vi "Lab Panel V5.10.vi"() -> ()   [LabVIEW 2013] (continued)
                                n574 = TDMS Open(6:FALSE, 10:T20."create or replace" ("operation (0:open)"), 11:w887) -> (0:w886:errorcluster, 3:→"TDMS LAB01-2":refnum<k34>)  [unwired: 4 in]
                              }
                              frame #2 {
                                n575 = local read "SET LAB01-2"() -> (w897:T5)
                                n576 = local read "TDMS LAB01-2"() -> (w908:refnum<k34>)
                                n577 = Build Array("Testers Name", "Description", "Set Test Cycles", "T-Rise minutes", "T-Rise Deg C") -> (w898:string[])
                                n578 = Unbundle(w897) -> ("NAME"=w896:string, "DESCRIPTION"=w895:string, "CYCLES"=w894:dbl, "T-RISE mins"=w893:dbl, "T-RISE deg C"=w892:dbl)
                                n579 = Number To Decimal String(number=w894) -> (decimal integer string=w907:string)  [unwired: 1 in]
                                n580 = Number To Decimal String(number=w893) -> (decimal integer string=w906:string)  [unwired: 1 in]
                                n581 = Number To Decimal String(number=w892) -> (decimal integer string=w905:string)  [unwired: 1 in]
                                n582 = Build Array(w896, w895, w907, w906, w905) -> (w904:string[])
                                n583 = TDMS Set Properties(5:w904, 7:w898, 11:w908) -> ()  [unwired: 3 in, 4 out]
                              }
                              frame #3 {
                                n584 = local read "DISP LAB01-2"() -> (w910:T4)
                                n585 = Concatenate Strings("LAB01-2  ", w913) -> (w914:string)
                                n586 = Two Button Dialog(message=w914, 1:w911, 2:w912) -> (T button?=w916:bool)
                                n587 = case shown="True" w916 {
                                tunnel: w910 -> [w923 w924]
                                tunnel: [w923 w924] -> w920
                                tunnel: [w922 w925] -> w919
                                tunnel: [w921 w925] -> w918
                                frame False {
                                n588 = Unbundle(w923) -> ("CYCLE"=w922:dbl, "MINS"=w921:dbl)  [unwired: 1 out]
                                }
                                frame True {
                                w925 = 0.0
                                }
                                }
                                n589 = Bundle(cluster=w920, "CYCLE"=w919, "MINS"=w918, "STATUS"="RUN") -> (w909:T4)
                                n590 = local write "DISP LAB01-2"(w909) -> ()
                              }
                              frame #4 {
                                n591 = local read "TEMP START LAB01-2"() -> (w928:cluster{"TL":dbl, "TN":dbl})
                                n592 = Bundle(cluster=w928, "TL"=w926, "TN"=w926) -> (w927:cluster{"TL":dbl, "TN":dbl})
                                n593 = local write "TEMP START LAB01-2"(w927) -> ()
                              }
                            }
                          }
                        }
                      }
                    }
                  }
                }
              }
              event "RUN LAB02-1": Value Change {
                n594 = event-data() -> ("NewVal"=w934:bool)  [unwired: 1 in, 5 out]
                n595 = local read "SIG LAB02-1"() -> (w930:T2)
                n596 = case shown="True" w934 {
                  tunnel: w940 -> [_ w978]
                  tunnel: w939 -> [_ w977]
                  tunnel: w937 -> [w942 w976]
                  tunnel: w938 -> [_ w975]
                  tunnel: w936 -> [_ w974]
                  tunnel: [w941 w973] -> w935
                  tunnel: w933 -> [_ w972]
                  tunnel: w932 -> [_ w971]
                  tunnel: w931 -> [_ w970]
                  tunnel: w930 -> [_ w969]
                  tunnel: w929 -> [_ w968]
                  frame False {
                    # "stop test"
                    n597 = stacked-sequence {
                      tunnel: w942 -> [w951 _]
                      tunnel: [w943 _] -> w941
                      frame #0 {
                        n598 = local read "DISP LAB02-1"() -> (w950:T4)
                        n599 = Unbundle(w950) -> ("CYCLE"=w948:dbl, "MINS"=w949:dbl)  [unwired: 1 out]
                        n600 = case shown="\"CYCLE TEST\"" w951 {
                          tunnel: w949 -> [_ _ w958]
                          tunnel: w948 -> [w956 w957 _]
                          tunnel: [w956 w957 w958] -> w947
                          frame "CHART TEST", Default {
                          }
                          frame "CYCLE TEST" {
                          }
                          frame "T-RISE TEST" {
                          }
                        }
                        n601 = local read "TDMS LAB02-1"() -> (w955:refnum<k34>)
                        n602 = Build Array("STOPPED") -> (w952:string[])
                        n603 = Build Array(w947) -> (w946:dbl[])
                        n604 = TDMS Write(0:w955, 5:"TEST RESULT", 7:w952, 9:w946) -> (4:w944:refnum<k34>, 15:w945:errorcluster)  [unwired: 2 in, 2 out]
                        n605 = TDMS Close(8:w945, 11:w944) -> (0:w943:errorcluster)  [unwired: 1 out]
                      }
                      frame #1 {
                        n606 = local read "DISP LAB02-1"() -> (w962:T4)
                        n607 = stacked-sequence {
                          tunnel: "LAB02-1" -> [w964 w966]
                          frame #0 {
                            n608 = call "sub vi - defrag tdms v1.vi"("panel id"=w964) -> ("error out"=w963:errorcluster)  [unwired: 10 in]
                            n609 = local write "data file error"(w963) -> ()
                          }
                          frame #1 {
                            n610 = local write "RESULT LAB02-1"(FALSE) -> ()
                            n611 = call "Save data file (stop) v3.vi"("panel id"=w966) -> ("network file save error"=w965:errorcluster)  [unwired: 9 in, 1 out]
                            n612 = local write "data file error"(w965) -> ()
                          }
                        }
                        n613 = Bundle(cluster=w962, "STATUS"="STOP") -> (w960:T4)  [unwired: 2 in]
                        n614 = local write "DISP LAB02-1"(w960) -> ()
                      }
                    }
                  }
                  frame True {
                    n615 = stacked-sequence {
                      seq-local: [w980 _] -> [_ w984]
                      tunnel: w978 -> [_ w994]
                      tunnel: w977 -> [_ w993]
                      tunnel: w976 -> [_ w992]
                      tunnel: w975 -> [_ w991]
                      tunnel: w974 -> [_ w990]
                      tunnel: [_ w989] -> w973
                      tunnel: w972 -> [_ w988]
                      tunnel: w971 -> [_ w987]
                      tunnel: w970 -> [_ w986]
                      tunnel: w969 -> [w979 w985]
                      tunnel: w968 -> [_ w983]
                      frame #0 {
                        n616 = Unbundle(w979) -> ("AMPS"=w982:dbl)  [unwired: 4 out]
                        n617 = call "Check For Amps on v1.vi"("ID"="LAB02-1", "amps"=w982) -> ("amps"=w980:bool)  [unwired: 9 in]
                      }
                      frame #1 {
                        n618 = case shown="True" w984 {
                          tunnel: w994 -> [_ w1007]
                          tunnel: w993 -> [_ w1006]
                          tunnel: w992 -> [_ w1005]
                          tunnel: w991 -> [_ w1004]
                          tunnel: w990 -> [_ w1003]
                          tunnel: [errorcluster {"status"=FALSE, "code"=0, "source"=""} ("error out") w1002] -> w989
                          tunnel: w988 -> [_ w1001]
                          tunnel: w987 -> [_ w1000]
                          tunnel: w986 -> [_ w999]
                          tunnel: w985 -> [_ w998]
                          tunnel: w983 -> [_ w997]
                          frame False {
                            w996 = FALSE
                            n619 = local write "RUN LAB02-1"(w996) -> ()
                            n620 = local write "run lab02-1"(w996) -> ()
                          }
                          frame True {
                            n621 = stacked-sequence {
                              seq-local: [w1008 _ _ _ _] -> [_ w1032 _ _ _]
                              tunnel: w1007 -> [w1013 _ _ _ _]
                              tunnel: w1006 -> [w1010 _ _ _ _]
                              tunnel: w1005 -> [w1023 _ _ _ _]
                              tunnel: w1004 -> [w1016 _ _ _ _]
                              tunnel: w1003 -> [w1011 _ _ _ _]
                              tunnel: [_ w1027 _ _ _] -> w1002
                              tunnel: w1001 -> [_ _ _ w1053 _]
                              tunnel: w1000 -> [_ _ _ w1052 _]
                              tunnel: w999 -> [_ _ _ w1051 _]
                              tunnel: w998 -> [_ _ _ _ _]
                              tunnel: w997 -> [_ _ _ _ w1067]
                              frame #0 {
                                w1009 = "\\"
                                n622 = local read "SET LAB02-1"() -> (w1018:T5)
                                n623 = case shown="\"CYCLE TEST\"" w1023 {
                                tunnel: ["L02-1-CHART TEST-" "L02-1-CYCLE TEST-" "L02-1-T-RISE TEST-"] -> w1019
                                frame "CHART TEST", Default {
                                }
                                frame "CYCLE TEST" {
                                }
                                frame "T-RISE TEST" {
                                }
                                }
                                n624 = Unbundle(w1018) -> ("DESCRIPTION"=w1017:string)  [unwired: 4 out]
                                n625 = Concatenate Strings(w1013, "\\", w1011, w1009, w1010, w1009) -> (w1020:string)
                                n626 = String To Path(string=w1020) -> (path=w1022:path)
                                n627 = Concatenate Strings(w1020, w1019, w1017, "-", w1016, ".tdms") -> (w1008:string)
                                n628 = Create Folder(path (use dialog)=w1022) -> (error out=w1021:errorcluster)  [unwired: 2 in, 2 out]
                                n629 = global write "Global 1.vi" "LAB02-1 FILE"(w1008) -> ()
                                n630 = call <vilib>:"Clear Errors.vi"("error in (no error)"=w1021) -> ()  [unwired: 6 in, 1 out]
                              }
                              frame #1 {
                                (unwired) FALSE
                                n631 = String To Path(string=w1032) -> (path=w1028:path)
                                n632 = TDMS Open(6:FALSE, 10:T20."create or replace" ("operation (0:open)"), 11:w1028) -> (0:w1027:errorcluster, 3:→"TDMS LAB02-1":refnum<k34>)  [unwired: 4 in]
                              }
                              frame #2 {
                                n633 = local read "SET LAB02-1"() -> (w1038:T5)
                                n634 = local read "TDMS LAB02-1"() -> (w1049:refnum<k34>)
                                n635 = Build Array("Testers Name", "Description", "Set Test Cycles", "T-Rise minutes", "T-Rise Deg C") -> (w1039:string[])
                                n636 = Unbundle(w1038) -> ("NAME"=w1037:string, "DESCRIPTION"=w1036:string, "CYCLES"=w1035:dbl, "T-RISE mins"=w1034:dbl, "T-RISE deg C"=w1033:dbl)
                                n637 = Number To Decimal String(number=w1035) -> (decimal integer string=w1048:string)  [unwired: 1 in]
                                n638 = Number To Decimal String(number=w1034) -> (decimal integer string=w1047:string)  [unwired: 1 in]
                                n639 = Number To Decimal String(number=w1033) -> (decimal integer string=w1046:string)  [unwired: 1 in]
                                n640 = Build Array(w1037, w1036, w1048, w1047, w1046) -> (w1045:string[])
                                n641 = TDMS Set Properties(5:w1045, 7:w1039, 11:w1049) -> ()  [unwired: 3 in, 4 out]
                              }
                              frame #3 {
                                n642 = local read "DISP LAB02-1"() -> (w1054:T4)
                                n643 = Concatenate Strings("LAB02-1  ", w1053) -> (w1055:string)
                                n644 = Two Button Dialog(message=w1055, 1:w1051, 2:w1052) -> (T button?=w1057:bool)
                                n645 = case shown="True" w1057 {
                                tunnel: w1054 -> [w1064 w1065]
                                tunnel: [w1064 w1065] -> w1061
                                tunnel: [w1063 w1066] -> w1060
                                tunnel: [w1062 w1066] -> w1059
                                frame False {
                                n646 = Unbundle(w1064) -> ("CYCLE"=w1063:dbl, "MINS"=w1062:dbl)  [unwired: 1 out]
                                }
                                frame True {
                                w1066 = 0.0
                                }
                                }
                                n647 = Bundle(cluster=w1061, "CYCLE"=w1060, "MINS"=w1059, "STATUS"="RUN") -> (w1050:T4)
                                n648 = local write "DISP LAB02-1"(w1050) -> ()
                              }
                              frame #4 {
                                n649 = local read "TEMP START LAB02-1"() -> (w1069:cluster{"TL":dbl, "TN":dbl})
                                n650 = Bundle(cluster=w1069, "TL"=w1067, "TN"=w1067) -> (w1068:cluster{"TL":dbl, "TN":dbl})
                                n651 = local write "TEMP START LAB02-1"(w1068) -> ()
                              }
                            }
                          }
                        }
                      }
                    }
                  }
                }
                n652 = local write "run lab02-1"(w934) -> ()
              }
              event "RUN LAB02-2": Value Change {
                n653 = event-data() -> ("NewVal"=w1074:bool)  [unwired: 1 in, 5 out]
                n654 = local write "run lab02-2"(w1074) -> ()
                n655 = case shown="True" w1074 {
                  tunnel: w1080 -> [_ w1118]
                  tunnel: w1079 -> [_ w1117]
                  tunnel: w1077 -> [w1082 w1116]
                  tunnel: w1078 -> [_ w1115]
                  tunnel: w1076 -> [_ w1114]
                  tunnel: [w1081 w1113] -> w1075
                  tunnel: w1073 -> [_ w1112]
                  tunnel: w1072 -> [_ w1111]
                  tunnel: w1071 -> [_ w1110]
                  tunnel: w1070 -> [_ w1108]
                  frame False {
                    # "stop test"
                    n656 = stacked-sequence {
                      tunnel: w1082 -> [w1091 _]
                      tunnel: [w1083 _] -> w1081
                      frame #0 {
                        n657 = local read "DISP LAB02-2"() -> (w1090:T4)
                        n658 = Unbundle(w1090) -> ("CYCLE"=w1088:dbl, "MINS"=w1089:dbl)  [unwired: 1 out]
                        n659 = case shown="\"CYCLE TEST\"" w1091 {
                          tunnel: w1089 -> [_ _ w1098]
                          tunnel: w1088 -> [w1096 w1097 _]
                          tunnel: [w1096 w1097 w1098] -> w1087
                          frame "CHART TEST", Default {
                          }
                          frame "CYCLE TEST" {
                          }
                          frame "T-RISE TEST" {
                          }
                        }
                        n660 = local read "TDMS LAB02-2"() -> (w1095:refnum<k34>)
                        n661 = Build Array("STOPPED") -> (w1092:string[])
                        n662 = Build Array(w1087) -> (w1086:dbl[])
                        n663 = TDMS Write(0:w1095, 5:"TEST RESULT", 7:w1092, 9:w1086) -> (4:w1084:refnum<k34>, 15:w1085:errorcluster)  [unwired: 2 in, 2 out]
                        n664 = TDMS Close(8:w1085, 11:w1084) -> (0:w1083:errorcluster)  [unwired: 1 out]
                      }
                      frame #1 {
                        n665 = local read "DISP LAB02-2"() -> (w1102:T4)
                        n666 = stacked-sequence {
                          tunnel: "LAB02-2" -> [w1104 w1106]
                          frame #0 {
                            n667 = call "sub vi - defrag tdms v1.vi"("panel id"=w1104) -> ("error out"=w1103:errorcluster)  [unwired: 10 in]
                            n668 = local write "data file error"(w1103) -> ()
                          }
                          frame #1 {
                            n669 = call "Save data file (stop) v3.vi"("panel id"=w1106) -> ("network file save error"=w1105:errorcluster)  [unwired: 9 in, 1 out]
                            n670 = local write "RESULT LAB02-2"(FALSE) -> ()
                            n671 = local write "data file error"(w1105) -> ()
                          }
                        }
                        n672 = Bundle(cluster=w1102, "STATUS"="STOP") -> (w1100:T4)  [unwired: 2 in]
                        n673 = local write "DISP LAB02-2"(w1100) -> ()
                      }
                    }
                  }
                  frame True {
                    n674 = local read "SIG LAB02-2"() -> (w1109:T2)
                    n675 = stacked-sequence {
                      seq-local: [w1120 _] -> [_ w1124]
                      tunnel: w1118 -> [_ w1134]
                      tunnel: w1117 -> [_ w1133]
                      tunnel: w1116 -> [_ w1132]
                      tunnel: w1115 -> [_ w1131]
                      tunnel: w1114 -> [_ w1130]
                      tunnel: [_ w1129] -> w1113
                      tunnel: w1112 -> [_ w1128]
                      tunnel: w1111 -> [_ w1127]
                      tunnel: w1110 -> [_ w1126]
                      tunnel: w1109 -> [w1119 w1125]
                      tunnel: w1108 -> [_ w1123]
                      frame #0 {
                        n676 = Unbundle(w1119) -> ("AMPS"=w1122:dbl)  [unwired: 4 out]
                        n677 = call "Check For Amps on v1.vi"("ID"="LAB02-2", "amps"=w1122) -> ("amps"=w1120:bool)  [unwired: 9 in]
                      }
                      frame #1 {
                        n678 = case shown="True" w1124 {
                          tunnel: w1134 -> [_ w1147]
                          tunnel: w1133 -> [_ w1146]
                          tunnel: w1132 -> [_ w1145]
                          tunnel: w1131 -> [_ w1144]
                          tunnel: w1130 -> [_ w1143]
                          tunnel: [errorcluster {"status"=FALSE, "code"=0, "source"=""} ("error out") w1142] -> w1129
                          tunnel: w1128 -> [_ w1141]
                          tunnel: w1127 -> [_ w1140]
                          tunnel: w1126 -> [_ w1139]
                          tunnel: w1125 -> [_ w1138]
                          tunnel: w1123 -> [_ w1137]
                          frame False {
                            w1135 = FALSE
                            n679 = local write "RUN LAB02-2"(w1135) -> ()
                            n680 = local write "run lab02-2"(w1135) -> ()
                          }
                          frame True {
                            n681 = stacked-sequence {
                              seq-local: [w1148 _ _ _ _] -> [_ w1172 _ _ _]
                              tunnel: w1147 -> [w1153 _ _ _ _]
                              tunnel: w1146 -> [w1150 _ _ _ _]
                              tunnel: w1145 -> [w1163 _ _ _ _]
                              tunnel: w1144 -> [w1156 _ _ _ _]
                              tunnel: w1143 -> [w1151 _ _ _ _]
                              tunnel: [_ w1167 _ _ _] -> w1142
                              tunnel: w1141 -> [_ _ _ w1193 _]
                              tunnel: w1140 -> [_ _ _ w1192 _]
                              tunnel: w1139 -> [_ _ _ w1191 _]
                              tunnel: w1138 -> [_ _ _ _ _]
                              tunnel: w1137 -> [_ _ _ _ w1207]
                              frame #0 {
                                w1149 = "\\"
                                n682 = local read "SET LAB02-2"() -> (w1158:T5)
                                n683 = case shown="\"CYCLE TEST\"" w1163 {
                                tunnel: ["L02-2-CHART TEST-" "L02-2-CYCLE TEST-" "L02-2-T-RISE TEST-"] -> w1159
                                frame "CHART TEST", Default {
                                }
                                frame "CYCLE TEST" {
                                }
                                frame "T-RISE TEST" {
                                }
                                }
                                n684 = Unbundle(w1158) -> ("DESCRIPTION"=w1157:string)  [unwired: 4 out]
                                n685 = Concatenate Strings(w1153, "\\", w1151, w1149, w1150, w1149) -> (w1160:string)
                                n686 = String To Path(string=w1160) -> (path=w1162:path)
                                n687 = Concatenate Strings(w1160, w1159, w1157, "-", w1156, ".tdms") -> (w1148:string)
                                n688 = Create Folder(path (use dialog)=w1162) -> (error out=w1161:errorcluster)  [unwired: 2 in, 2 out]
                                n689 = global write "Global 1.vi" "LAB02-2 FILE"(w1148) -> ()
                                n690 = call <vilib>:"Clear Errors.vi"("error in (no error)"=w1161) -> ()  [unwired: 6 in, 1 out]
                              }
                              frame #1 {
                                (unwired) FALSE
                                n691 = String To Path(string=w1172) -> (path=w1168:path)
                                n692 = TDMS Open(6:FALSE, 10:T20."create or replace" ("operation (0:open)"), 11:w1168) -> (0:w1167:errorcluster, 3:→"TDMS LAB02-2":refnum<k34>)  [unwired: 4 in]
                              }
                              frame #2 {
                                n693 = local read "SET LAB02-2"() -> (w1178:T5)
                                n694 = local read "TDMS LAB02-2"() -> (w1189:refnum<k34>)
                                n695 = Build Array("Testers Name", "Description", "Set Test Cycles", "T-Rise minutes", "T-Rise Deg C") -> (w1179:string[])
                                n696 = Unbundle(w1178) -> ("NAME"=w1177:string, "DESCRIPTION"=w1176:string, "CYCLES"=w1175:dbl, "T-RISE mins"=w1174:dbl, "T-RISE deg C"=w1173:dbl)
                                n697 = Number To Decimal String(number=w1175) -> (decimal integer string=w1188:string)  [unwired: 1 in]
                                n698 = Number To Decimal String(number=w1174) -> (decimal integer string=w1187:string)  [unwired: 1 in]
                                n699 = Number To Decimal String(number=w1173) -> (decimal integer string=w1186:string)  [unwired: 1 in]
                                n700 = Build Array(w1177, w1176, w1188, w1187, w1186) -> (w1185:string[])
                                n701 = TDMS Set Properties(5:w1185, 7:w1179, 11:w1189) -> ()  [unwired: 3 in, 4 out]
                              }
                              frame #3 {
                                n702 = local read "DISP LAB02-2"() -> (w1194:T4)
                                n703 = Concatenate Strings("LAB02-2  ", w1193) -> (w1195:string)
                                n704 = Two Button Dialog(message=w1195, 1:w1191, 2:w1192) -> (T button?=w1197:bool)
                                n705 = case shown="True" w1197 {
                                tunnel: w1194 -> [w1204 w1205]
                                tunnel: [w1204 w1205] -> w1201
                                tunnel: [w1203 w1206] -> w1200
                                tunnel: [w1202 w1206] -> w1199
                                frame False {
                                n706 = Unbundle(w1204) -> ("CYCLE"=w1203:dbl, "MINS"=w1202:dbl)  [unwired: 1 out]
                                }
                                frame True {
                                w1206 = 0.0
                                }
                                }
                                n707 = Bundle(cluster=w1201, "CYCLE"=w1200, "MINS"=w1199, "STATUS"="RUN") -> (w1190:T4)
                                n708 = local write "DISP LAB02-2"(w1190) -> ()
                              }
                              frame #4 {
                                n709 = local read "TEMP START LAB02-2"() -> (w1209:cluster{"TL":dbl, "TN":dbl})
                                n710 = Bundle(cluster=w1209, "TL"=w1207, "TN"=w1207) -> (w1208:cluster{"TL":dbl, "TN":dbl})
                                n711 = local write "TEMP START LAB02-2"(w1208) -> ()
                              }
                            }
                          }
                        }
                      }
                    }
                  }
                }
              }
              event "RUN LAB03-1": Value Change {
                n712 = event-data() -> ("NewVal"=w1214:bool)  [unwired: 1 in, 5 out]
                n713 = local write "run lab03-1"(w1214) -> ()
                n714 = case shown="True" w1214 {
                  tunnel: w1220 -> [_ w1258]
                  tunnel: w1219 -> [_ w1257]
                  tunnel: w1217 -> [w1222 w1256]
                  tunnel: w1218 -> [_ w1255]
                  tunnel: w1216 -> [_ w1254]
                  tunnel: [w1221 w1253] -> w1215
                  tunnel: w1213 -> [_ w1252]
                  tunnel: w1212 -> [_ w1251]
                  tunnel: w1211 -> [_ w1250]
                  tunnel: w1210 -> [_ w1248]
                  frame False {
                    # "stop test"
                    n715 = stacked-sequence {
                      tunnel: w1222 -> [w1231 _]
                      tunnel: [w1223 _] -> w1221
                      frame #0 {
                        n716 = local read "DISP LAB03-1"() -> (w1230:T4)
                        n717 = Unbundle(w1230) -> ("CYCLE"=w1228:dbl, "MINS"=w1229:dbl)  [unwired: 1 out]
                        n718 = case shown="\"CYCLE TEST\"" w1231 {
                          tunnel: w1229 -> [_ _ w1238]
                          tunnel: w1228 -> [w1236 w1237 _]
                          tunnel: [w1236 w1237 w1238] -> w1227
                          frame "CHART TEST", Default {
                          }
                          frame "CYCLE TEST" {
                          }
                          frame "T-RISE TEST" {
                          }
                        }
                        n719 = local read "TDMS LAB03-1"() -> (w1235:refnum<k34>)
                        n720 = Build Array("STOPPED") -> (w1232:string[])
                        n721 = Build Array(w1227) -> (w1226:dbl[])
                        n722 = TDMS Write(0:w1235, 5:"TEST RESULT", 7:w1232, 9:w1226) -> (4:w1224:refnum<k34>, 15:w1225:errorcluster)  [unwired: 2 in, 2 out]
                        n723 = TDMS Close(8:w1225, 11:w1224) -> (0:w1223:errorcluster)  [unwired: 1 out]
                      }
                      frame #1 {
                        n724 = local read "DISP LAB03-1"() -> (w1242:T4)
                        n725 = stacked-sequence {
                          tunnel: "LAB03-1" -> [w1244 w1246]
                          frame #0 {
                            n726 = call "sub vi - defrag tdms v1.vi"("panel id"=w1244) -> ("error out"=w1243:errorcluster)  [unwired: 10 in]
                            n727 = local write "data file error"(w1243) -> ()
                          }
                          frame #1 {
                            n728 = call "Save data file (stop) v3.vi"("panel id"=w1246) -> ("network file save error"=w1245:errorcluster)  [unwired: 9 in, 1 out]
                            n729 = local write "RESULT LAB03-1"(FALSE) -> ()
                            n730 = local write "data file error"(w1245) -> ()
                          }
                        }
                        n731 = Bundle(cluster=w1242, "STATUS"="STOP") -> (w1240:T4)  [unwired: 2 in]
                        n732 = local write "DISP LAB03-1"(w1240) -> ()
                      }
                    }
                  }
                  frame True {
                    n733 = local read "SIG LAB03-1"() -> (w1249:T2)
                    n734 = stacked-sequence {
                      seq-local: [w1260 _] -> [_ w1264]
                      tunnel: w1258 -> [_ w1274]
                      tunnel: w1257 -> [_ w1273]
                      tunnel: w1256 -> [_ w1272]
                      tunnel: w1255 -> [_ w1271]
                      tunnel: w1254 -> [_ w1270]
                      tunnel: [_ w1269] -> w1253
                      tunnel: w1252 -> [_ w1268]
                      tunnel: w1251 -> [_ w1267]
                      tunnel: w1250 -> [_ w1266]
                      tunnel: w1249 -> [w1259 w1265]
                      tunnel: w1248 -> [_ w1263]
                      frame #0 {
                        n735 = Unbundle(w1259) -> ("AMPS"=w1262:dbl)  [unwired: 4 out]
                        n736 = call "Check For Amps on v1.vi"("ID"="LAB03-1", "amps"=w1262) -> ("amps"=w1260:bool)  [unwired: 9 in]
                      }
                      frame #1 {
                        n737 = case shown="True" w1264 {
                          tunnel: w1274 -> [_ w1287]
                          tunnel: w1273 -> [_ w1286]
                          tunnel: w1272 -> [_ w1285]
                          tunnel: w1271 -> [_ w1284]
                          tunnel: w1270 -> [_ w1283]
                          tunnel: [errorcluster {"status"=FALSE, "code"=0, "source"=""} ("error out") w1282] -> w1269
                          tunnel: w1268 -> [_ w1281]
                          tunnel: w1267 -> [_ w1280]
                          tunnel: w1266 -> [_ w1279]
                          tunnel: w1265 -> [_ w1278]
                          tunnel: w1263 -> [_ w1277]
                          frame False {
                            w1275 = FALSE
                            n738 = local write "RUN LAB03-1"(w1275) -> ()
                            n739 = local write "run lab03-1"(w1275) -> ()
                          }
                          frame True {
                            n740 = stacked-sequence {
                              seq-local: [w1288 _ _ _ _] -> [_ w1312 _ _ _]
                              tunnel: w1287 -> [w1293 _ _ _ _]
                              tunnel: w1286 -> [w1290 _ _ _ _]
                              tunnel: w1285 -> [w1303 _ _ _ _]
                              tunnel: w1284 -> [w1296 _ _ _ _]
                              tunnel: w1283 -> [w1291 _ _ _ _]
                              tunnel: [_ w1307 _ _ _] -> w1282
                              tunnel: w1281 -> [_ _ _ w1332 _]
                              tunnel: w1280 -> [_ _ _ w1331 _]
                              tunnel: w1279 -> [_ _ _ w1330 _]
                              tunnel: w1278 -> [_ _ _ _ _]
                              tunnel: w1277 -> [_ _ _ _ w1347]
                              frame #0 {
                                w1289 = "\\"
                                n741 = local read "SET LAB03-1"() -> (w1298:T5)
                                n742 = case shown="\"T-RISE TEST\"" w1303 {
                                tunnel: ["L03-1-CHART TEST-" "L03-1-CYCLE TEST-" "L03-1-T-RISE TEST-"] -> w1299
                                frame "CHART TEST", Default {
                                }
                                frame "CYCLE TEST" {
                                }
                                frame "T-RISE TEST" {
                                }
                                }
                                n743 = Unbundle(w1298) -> ("DESCRIPTION"=w1297:string)  [unwired: 4 out]
                                n744 = Concatenate Strings(w1293, "\\", w1291, w1289, w1290, w1289) -> (w1300:string)
                                n745 = String To Path(string=w1300) -> (path=w1302:path)
                                n746 = Concatenate Strings(w1300, w1299, w1297, "-", w1296, ".tdms") -> (w1288:string)
                                n747 = Create Folder(path (use dialog)=w1302) -> (error out=w1301:errorcluster)  [unwired: 2 in, 2 out]
                                n748 = global write "Global 1.vi" "LAB03-1 FILE"(w1288) -> ()
                                n749 = call <vilib>:"Clear Errors.vi"("error in (no error)"=w1301) -> ()  [unwired: 6 in, 1 out]
                              }
                              frame #1 {
                                (unwired) FALSE
                                n750 = String To Path(string=w1312) -> (path=w1308:path)
                                n751 = TDMS Open(6:FALSE, 10:T20."create or replace" ("operation (0:open)"), 11:w1308) -> (0:w1307:errorcluster, 3:→"TDMS LAB03-1":refnum<k34>)  [unwired: 4 in]
                              }
                              frame #2 {
                                n752 = local read "SET LAB03-1"() -> (w1318:T5)
                                n753 = local read "TDMS LAB03-1"() -> (w1329:refnum<k34>)
                                n754 = Build Array("Testers Name", "Description", "Set Test Cycles", "T-Rise minutes", "T-Rise Deg C") -> (w1319:string[])
                                n755 = Unbundle(w1318) -> ("NAME"=w1317:string, "DESCRIPTION"=w1316:string, "CYCLES"=w1315:dbl, "T-RISE mins"=w1314:dbl, "T-RISE deg C"=w1313:dbl)
                                n756 = Number To Decimal String(number=w1315) -> (decimal integer string=w1328:string)  [unwired: 1 in]
                                n757 = Number To Decimal String(number=w1314) -> (decimal integer string=w1327:string)  [unwired: 1 in]
                                n758 = Number To Decimal String(number=w1313) -> (decimal integer string=w1326:string)  [unwired: 1 in]
                                n759 = Build Array(w1317, w1316, w1328, w1327, w1326) -> (w1325:string[])
                                n760 = TDMS Set Properties(5:w1325, 7:w1319, 11:w1329) -> ()  [unwired: 3 in, 4 out]
                              }
                              frame #3 {
                                n761 = local read "DISP LAB03-1"() -> (w1334:T4)
                                n762 = Concatenate Strings("LAB03-1  ", w1332) -> (w1335:string)
                                n763 = Two Button Dialog(message=w1335, 1:w1330, 2:w1331) -> (T button?=w1337:bool)
                                n764 = case shown="True" w1337 {
                                tunnel: w1334 -> [w1344 w1345]
                                tunnel: [w1344 w1345] -> w1341
                                tunnel: [w1343 w1346] -> w1340
                                tunnel: [w1342 w1346] -> w1339
                                frame False {
                                n765 = Unbundle(w1344) -> ("CYCLE"=w1343:dbl, "MINS"=w1342:dbl)  [unwired: 1 out]
                                }
                                frame True {
                                w1346 = 0.0
                                }
                                }
                                n766 = Bundle(cluster=w1341, "CYCLE"=w1340, "MINS"=w1339, "STATUS"="RUN") -> (w1333:T4)
                                n767 = local write "DISP LAB03-1"(w1333) -> ()
                              }
                              frame #4 {
                                n768 = local read "TEMP START LAB03-1"() -> (w1349:cluster{"TL":dbl, "TN":dbl})
                                n769 = Bundle(cluster=w1349, "TL"=w1347, "TN"=w1347) -> (w1348:cluster{"TL":dbl, "TN":dbl})
                                n770 = local write "TEMP START LAB03-1"(w1348) -> ()
                              }
                            }
                          }
                        }
                      }
                    }
                  }
                }
              }
              event "RUN LAB03-2": Value Change {
                n771 = event-data() -> ("NewVal"=w1354:bool)  [unwired: 1 in, 5 out]
                n772 = local write "run lab03-2"(w1354) -> ()
                n773 = case shown="True" w1354 {
                  tunnel: w1360 -> [_ w1398]
                  tunnel: w1359 -> [_ w1397]
                  tunnel: w1357 -> [w1362 w1396]
                  tunnel: w1358 -> [_ w1395]
                  tunnel: w1356 -> [_ w1394]
                  tunnel: [w1361 w1393] -> w1355
                  tunnel: w1353 -> [_ w1392]
                  tunnel: w1352 -> [_ w1391]
                  tunnel: w1351 -> [_ w1390]
                  tunnel: w1350 -> [_ w1388]
                  frame False {
                    # "stop test"
                    n774 = stacked-sequence {
                      tunnel: w1362 -> [w1371 _]
                      tunnel: [w1363 _] -> w1361
                      frame #0 {
                        n775 = local read "DISP LAB03-2"() -> (w1370:T4)
                        n776 = Unbundle(w1370) -> ("CYCLE"=w1368:dbl, "MINS"=w1369:dbl)  [unwired: 1 out]
                        n777 = case shown="\"CYCLE TEST\"" w1371 {
                          tunnel: w1369 -> [_ _ w1378]
                          tunnel: w1368 -> [w1376 w1377 _]
                          tunnel: [w1376 w1377 w1378] -> w1367
                          frame "CHART TEST", Default {
                          }
                          frame "CYCLE TEST" {
                          }
                          frame "T-RISE TEST" {
                          }
                        }
                        n778 = local read "TDMS LAB03-2"() -> (w1375:refnum<k34>)
                        n779 = Build Array("STOPPED") -> (w1372:string[])
                        n780 = Build Array(w1367) -> (w1366:dbl[])
                        n781 = TDMS Write(0:w1375, 5:"TEST RESULT", 7:w1372, 9:w1366) -> (4:w1364:refnum<k34>, 15:w1365:errorcluster)  [unwired: 2 in, 2 out]
                        n782 = TDMS Close(8:w1365, 11:w1364) -> (0:w1363:errorcluster)  [unwired: 1 out]
                      }
                      frame #1 {
                        n783 = local read "DISP LAB03-2"() -> (w1382:T4)
                        n784 = stacked-sequence {
                          tunnel: "LAB03-2" -> [w1384 w1386]
                          frame #0 {
                            n785 = call "sub vi - defrag tdms v1.vi"("panel id"=w1384) -> ("error out"=w1383:errorcluster)  [unwired: 10 in]
                            n786 = local write "data file error"(w1383) -> ()
                          }
                          frame #1 {
                            n787 = call "Save data file (stop) v3.vi"("panel id"=w1386) -> ("network file save error"=w1385:errorcluster)  [unwired: 9 in, 1 out]
                            n788 = local write "RESULT LAB03-2"(FALSE) -> ()
                            n789 = local write "data file error"(w1385) -> ()
                          }
                        }
                        n790 = Bundle(cluster=w1382, "STATUS"="STOP") -> (w1380:T4)  [unwired: 2 in]
                        n791 = local write "DISP LAB03-2"(w1380) -> ()
                      }
                    }
                  }
                  frame True {
                    n792 = local read "SIG LAB03-2"() -> (w1389:T2)
                    n793 = stacked-sequence {
                      seq-local: [w1400 _] -> [_ w1404]
                      tunnel: w1398 -> [_ w1414]
                      tunnel: w1397 -> [_ w1413]
                      tunnel: w1396 -> [_ w1412]
                      tunnel: w1395 -> [_ w1411]
                      tunnel: w1394 -> [_ w1410]
                      tunnel: [_ w1409] -> w1393
                      tunnel: w1392 -> [_ w1408]
                      tunnel: w1391 -> [_ w1407]
                      tunnel: w1390 -> [_ w1406]
                      tunnel: w1389 -> [w1399 w1405]
                      tunnel: w1388 -> [_ w1403]
                      frame #0 {
                        n794 = Unbundle(w1399) -> ("AMPS"=w1402:dbl)  [unwired: 4 out]
                        n795 = call "Check For Amps on v1.vi"("ID"="LAB03-2", "amps"=w1402) -> ("amps"=w1400:bool)  [unwired: 9 in]
                      }
                      frame #1 {
                        n796 = case shown="True" w1404 {
                          tunnel: w1414 -> [_ w1427]
                          tunnel: w1413 -> [_ w1426]
                          tunnel: w1412 -> [_ w1425]
                          tunnel: w1411 -> [_ w1424]
                          tunnel: w1410 -> [_ w1423]
                          tunnel: [errorcluster {"status"=FALSE, "code"=0, "source"=""} ("error out") w1422] -> w1409
                          tunnel: w1408 -> [_ w1421]
                          tunnel: w1407 -> [_ w1420]
                          tunnel: w1406 -> [_ w1419]
                          tunnel: w1405 -> [_ w1418]
                          tunnel: w1403 -> [_ w1417]
                          frame False {
                            w1415 = FALSE
                            n797 = local write "RUN LAB03-2"(w1415) -> ()
                            n798 = local write "run lab03-2"(w1415) -> ()
                          }
                          frame True {
                            n799 = stacked-sequence {
                              seq-local: [w1428 _ _ _ _] -> [_ w1452 _ _ _]
                              tunnel: w1427 -> [w1433 _ _ _ _]
                              tunnel: w1426 -> [w1430 _ _ _ _]
                              tunnel: w1425 -> [w1443 _ _ _ _]
                              tunnel: w1424 -> [w1436 _ _ _ _]
                              tunnel: w1423 -> [w1431 _ _ _ _]
                              tunnel: [_ w1447 _ _ _] -> w1422
                              tunnel: w1421 -> [_ _ _ w1473 _]
                              tunnel: w1420 -> [_ _ _ w1472 _]
                              tunnel: w1419 -> [_ _ _ w1471 _]
                              tunnel: w1418 -> [_ _ _ _ _]
                              tunnel: w1417 -> [_ _ _ _ w1487]
                              frame #0 {
                                w1429 = "\\"
                                n800 = local read "SET LAB03-2"() -> (w1438:T5)
                                n801 = case shown="\"T-RISE TEST\"" w1443 {
                                tunnel: ["L03-2-CHART TEST-" "L03-2-CYCLE TEST-" "L03-2-T-RISE TEST-"] -> w1439
                                frame "CHART TEST", Default {
                                }
                                frame "CYCLE TEST" {
                                }
                                frame "T-RISE TEST" {
                                }
                                }
                                n802 = Unbundle(w1438) -> ("DESCRIPTION"=w1437:string)  [unwired: 4 out]
                                n803 = Concatenate Strings(w1433, "\\", w1431, w1429, w1430, w1429) -> (w1440:string)
                                n804 = String To Path(string=w1440) -> (path=w1442:path)
                                n805 = Concatenate Strings(w1440, w1439, w1437, "-", w1436, ".tdms") -> (w1428:string)
                                n806 = Create Folder(path (use dialog)=w1442) -> (error out=w1441:errorcluster)  [unwired: 2 in, 2 out]
                                n807 = global write "Global 1.vi" "LAB03-2 FILE"(w1428) -> ()
                                n808 = call <vilib>:"Clear Errors.vi"("error in (no error)"=w1441) -> ()  [unwired: 6 in, 1 out]
                              }
                              frame #1 {
                                (unwired) FALSE
                                n809 = String To Path(string=w1452) -> (path=w1448:path)
                                n810 = TDMS Open(6:FALSE, 10:T20."create or replace" ("operation (0:open)"), 11:w1448) -> (0:w1447:errorcluster, 3:→"TDMS LAB03-2":refnum<k34>)  [unwired: 4 in]
                              }
                              frame #2 {
                                n811 = local read "SET LAB03-2"() -> (w1458:T5)
                                n812 = local read "TDMS LAB03-2"() -> (w1469:refnum<k34>)
                                n813 = Build Array("Testers Name", "Description", "Set Test Cycles", "T-Rise minutes", "T-Rise Deg C") -> (w1459:string[])
                                n814 = Unbundle(w1458) -> ("NAME"=w1457:string, "DESCRIPTION"=w1456:string, "CYCLES"=w1455:dbl, "T-RISE mins"=w1454:dbl, "T-RISE deg C"=w1453:dbl)
                                n815 = Number To Decimal String(number=w1455) -> (decimal integer string=w1468:string)  [unwired: 1 in]
                                n816 = Number To Decimal String(number=w1454) -> (decimal integer string=w1467:string)  [unwired: 1 in]
                                n817 = Number To Decimal String(number=w1453) -> (decimal integer string=w1466:string)  [unwired: 1 in]
                                n818 = Build Array(w1457, w1456, w1468, w1467, w1466) -> (w1465:string[])
                                n819 = TDMS Set Properties(5:w1465, 7:w1459, 11:w1469) -> ()  [unwired: 3 in, 4 out]
                              }
                              frame #3 {
                                n820 = local read "DISP LAB03-2"() -> (w1474:T4)
                                n821 = Concatenate Strings("LAB03-2  ", w1473) -> (w1475:string)
                                n822 = Two Button Dialog(message=w1475, 1:w1471, 2:w1472) -> (T button?=w1477:bool)
                                n823 = case shown="True" w1477 {
                                tunnel: w1474 -> [w1484 w1485]
                                tunnel: [w1484 w1485] -> w1481
                                tunnel: [w1483 w1486] -> w1480
                                tunnel: [w1482 w1486] -> w1479
                                frame False {
                                n824 = Unbundle(w1484) -> ("CYCLE"=w1483:dbl, "MINS"=w1482:dbl)  [unwired: 1 out]
                                }
                                frame True {
                                w1486 = 0.0
                                }
                                }
                                n825 = Bundle(cluster=w1481, "CYCLE"=w1480, "MINS"=w1479, "STATUS"="RUN") -> (w1470:T4)
                                n826 = local write "DISP LAB03-2"(w1470) -> ()
                              }
                              frame #4 {
                                n827 = local read "TEMP START LAB03-2"() -> (w1489:cluster{"TL":dbl, "TN":dbl})
                                n828 = Bundle(cluster=w1489, "TL"=w1487, "TN"=w1487) -> (w1488:cluster{"TL":dbl, "TN":dbl})
                                n829 = local write "TEMP START LAB03-2"(w1488) -> ()
                              }
                            }
                          }
                        }
                      }
                    }
                  }
                }
              }
              event "RUN LAB04-1": Value Change {
                n830 = event-data() -> ("NewVal"=w1494:bool)  [unwired: 1 in, 5 out]
                n831 = local write "run lab04-1"(w1494) -> ()
                n832 = case shown="True" w1494 {
                  tunnel: w1500 -> [_ w1538]
                  tunnel: w1499 -> [_ w1537]
                  tunnel: w1497 -> [w1502 w1536]
                  tunnel: w1498 -> [_ w1535]
                  tunnel: w1496 -> [_ w1534]
                  tunnel: [w1501 w1533] -> w1495
                  tunnel: w1493 -> [_ w1532]
                  tunnel: w1492 -> [_ w1531]
                  tunnel: w1491 -> [_ w1530]
                  tunnel: w1490 -> [_ w1528]
                  frame False {
                    # "stop test"
                    n833 = stacked-sequence {
                      tunnel: w1502 -> [w1511 _]
                      tunnel: [w1503 _] -> w1501
                      frame #0 {
                        n834 = local read "DISP LAB04-1"() -> (w1510:T4)
                        n835 = Unbundle(w1510) -> ("CYCLE"=w1508:dbl, "MINS"=w1509:dbl)  [unwired: 1 out]
                        n836 = case shown="\"CYCLE TEST\"" w1511 {
                          tunnel: w1509 -> [_ _ w1518]
                          tunnel: w1508 -> [w1516 w1517 _]
                          tunnel: [w1516 w1517 w1518] -> w1507
                          frame "CHART TEST", Default {
                          }
                          frame "CYCLE TEST" {
                          }
                          frame "T-RISE TEST" {
                          }
                        }
                        n837 = local read "TDMS LAB04-1"() -> (w1515:refnum<k34>)
                        n838 = Build Array("STOPPED") -> (w1512:string[])
                        n839 = Build Array(w1507) -> (w1506:dbl[])
                        n840 = TDMS Write(0:w1515, 5:"TEST RESULT", 7:w1512, 9:w1506) -> (4:w1504:refnum<k34>, 15:w1505:errorcluster)  [unwired: 2 in, 2 out]
                        n841 = TDMS Close(8:w1505, 11:w1504) -> (0:w1503:errorcluster)  [unwired: 1 out]
                      }
                      frame #1 {
                        n842 = local read "DISP LAB04-1"() -> (w1522:T4)
                        n843 = stacked-sequence {
                          tunnel: "LAB04-1" -> [w1524 w1526]
                          frame #0 {
                            n844 = call "sub vi - defrag tdms v1.vi"("panel id"=w1524) -> ("error out"=w1523:errorcluster)  [unwired: 10 in]
                            n845 = local write "data file error"(w1523) -> ()
                          }
                          frame #1 {
                            n846 = call "Save data file (stop) v3.vi"("panel id"=w1526) -> ("network file save error"=w1525:errorcluster)  [unwired: 9 in, 1 out]
                            n847 = local write "RESULT LAB04-1"(FALSE) -> ()
